vi "mapV3.vi"() -> ()   [LabVIEW 2024]
uses:
  D:/Autonomous Systems/Oulu/Measurment Systems/Examples/GMap.NET/GMapControl/GMapControl/bin/Debug/GMapControl.dll
  GMap.NET/GMapControl/GMapControl/bin/Debug/GMapControl.dll
panel:
  out "GetLongitude":dbl
  out "GetLatitude":dbl
  out "Button":u16
  out "mouse event":bool
  in  "MapControl":refnum<k24>(container)
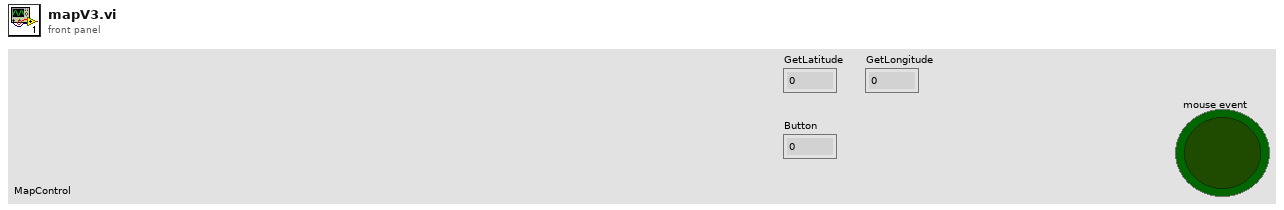
[diagram p1: front panel]
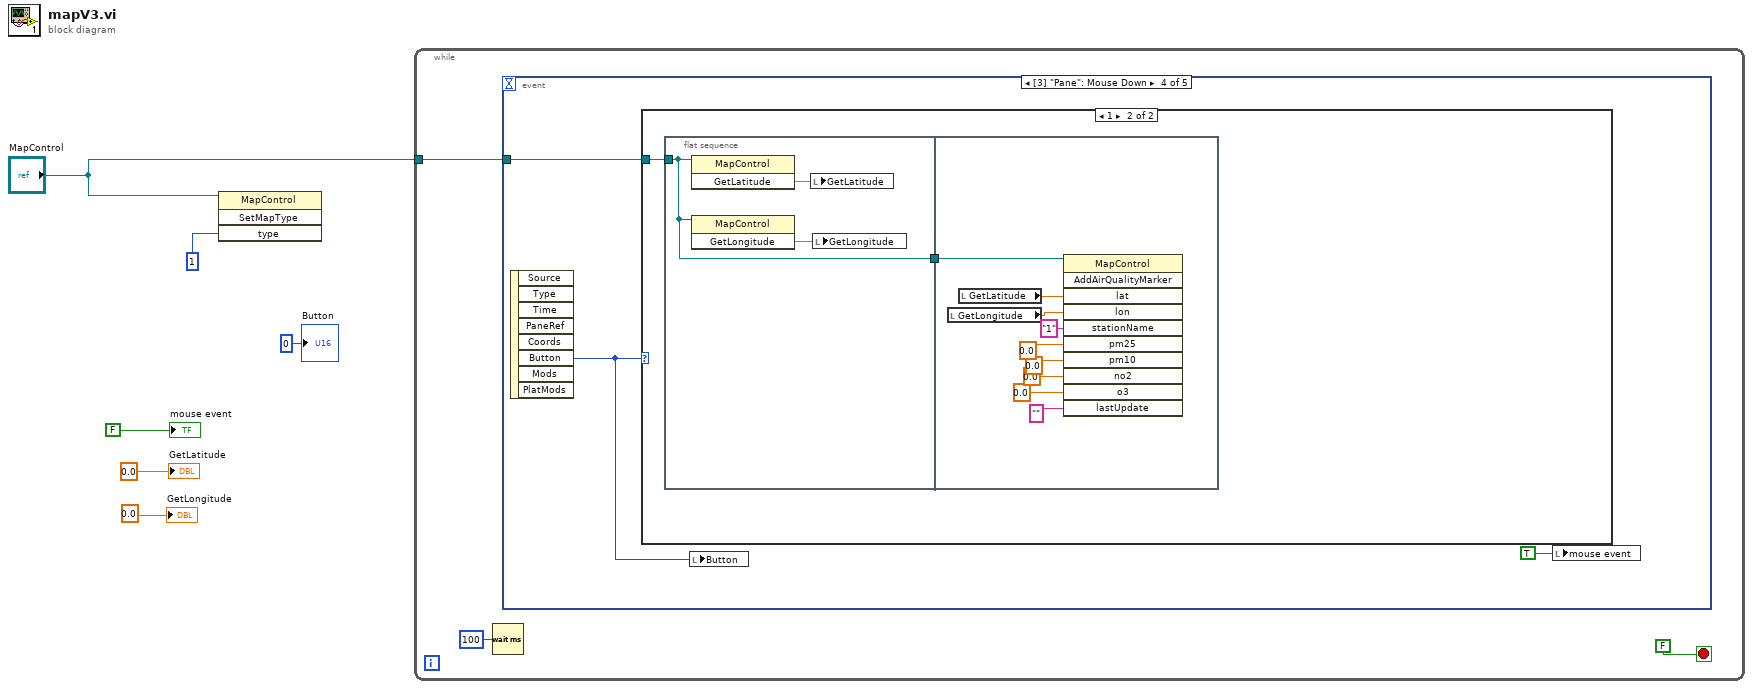
[diagram p0: block diagram]
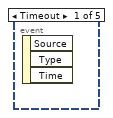
[diagram p2: hidden frame]
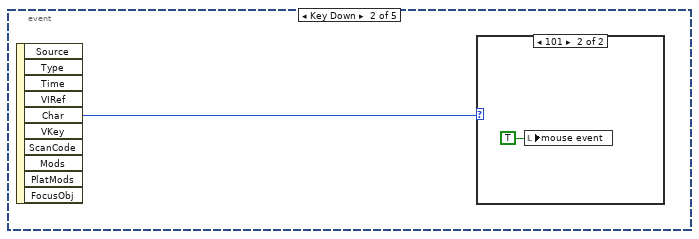
[diagram p3: hidden frame]
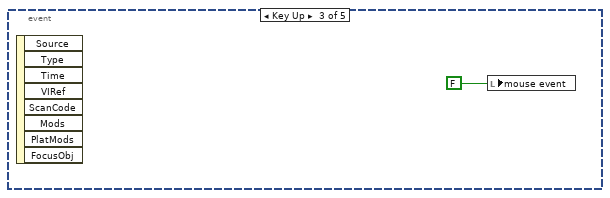
[diagram p5: hidden frame]
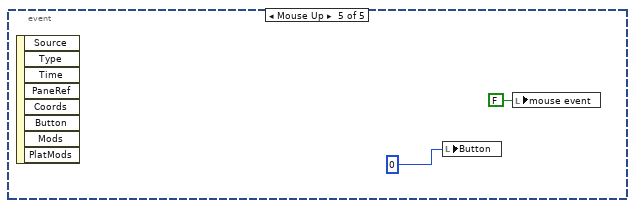
[diagram p7: hidden frame]
diagram:
  n1 = invoke class="MapControl" method="SetMapType"(reference="MapControl", "type"=1) -> ()  [unwired: 2 in, 4 out]
  n2 = while {
    tunnel: "MapControl" -> [w7]
    stop <- FALSE stop-if-true
    n3 = Wait (ms)(milliseconds to wait=u32 100) -> ()  [unwired: 1 out]
    n4 = event shown="[3] \"Pane\": Mouse Down" {
      selector: _ -> [_ _ _ _ _]
      dyn-events: _ -> [_ _ _ _ _]
      timeout: _ -> [_ _ _ _ _]
      tunnel: w7 -> [_ _ _ w14 _]
      event Timeout {
        n5 = event-data() -> ()  [unwired: 1 in, 3 out]
      }
      event Key Down {
        n6 = event-data() -> ("Char"=w10:i16)  [unwired: 1 in, 9 out]
        n7 = case shown="101" w10 {
          frame Default {
          }
          frame 101 {
            n8 = local write "mouse event"(TRUE ("mouse event")) -> ()
          }
        }
      }
      event Key Up {
        n9 = event-data() -> ()  [unwired: 1 in, 8 out]
        n10 = local write "mouse event"(FALSE ("mouse event")) -> ()
      }
      event Mouse Down {
        n11 = event-data() -> ("Button"=w13:u16)  [unwired: 1 in, 7 out]
        n12 = case shown="1" w13 {
          tunnel: w14 -> [_ w17]
          frame Default {
          }
          frame 1 {
            n13 = flat-sequence {
              tunnel: w17 -> [w18]
              tunnel: [w18] -> w16
              tunnel: w16 -> [w29]
              frame #0 {
                n14 = invoke class="MapControl" method="GetLatitude"(reference=w18) -> ("GetLatitude"=w20:dbl)  [unwired: 2 in, 2 out]
                n15 = invoke class="MapControl" method="GetLongitude"(reference=w18) -> ("GetLongitude"=w19:dbl)  [unwired: 2 in, 2 out]
                n16 = local write "GetLatitude"(w20) -> ()
                n17 = local write "GetLongitude"(w19) -> ()
              }
              frame #1 {
                n18 = local read "GetLongitude"() -> (w27:dbl)
                n19 = local read "GetLatitude"() -> (w28:dbl)
                n20 = invoke class="MapControl" method="AddAirQualityMarker"(reference=w29, "lat"=w28, "lon"=w27, "stationName"="1", "pm25"=0.0, "pm10"=0.0, "no2"=0.0, "o3"=0.0, "lastUpdate"="") -> ()  [unwired: 2 in, 11 out]
              }
            }
          }
        }
        n21 = local write "Button"(w13) -> ()
        n22 = local write "mouse event"(TRUE ("mouse event")) -> ()
      }
      event Mouse Up {
        n23 = event-data() -> ()  [unwired: 1 in, 8 out]
        n24 = local write "Button"(u16 0 ("Button")) -> ()
        n25 = local write "mouse event"(FALSE ("mouse event")) -> ()
      }
    }
  }
  "mouse event" <- FALSE ("mouse event")
  "Button" <- u16 0 ("Button")
  "GetLatitude" <- 0.0 ("GetLatitude")
  "GetLongitude" <- 0.0 ("GetLongitude")
